vi "Playing with Resources.vi"() -> ()   [LabVIEW 2012]
uses:
  _ResManager_v86/ID_Resource info.ctl
  _ResManager_v86/IDCloneResMgr.lvlib
panel:
  out "Array":string[](array[string])
  in  "resource binary file":path=path "C:/Users/Francois/SkyDrive/_DESIM/Projets/UI Tools Addons/UI Tools Control Class/ctl_class/Templates/System vectoriel.ctl"
  out "resources":T1[](array[typedef]) {"type" format="%.0x"}
  out "file type":string
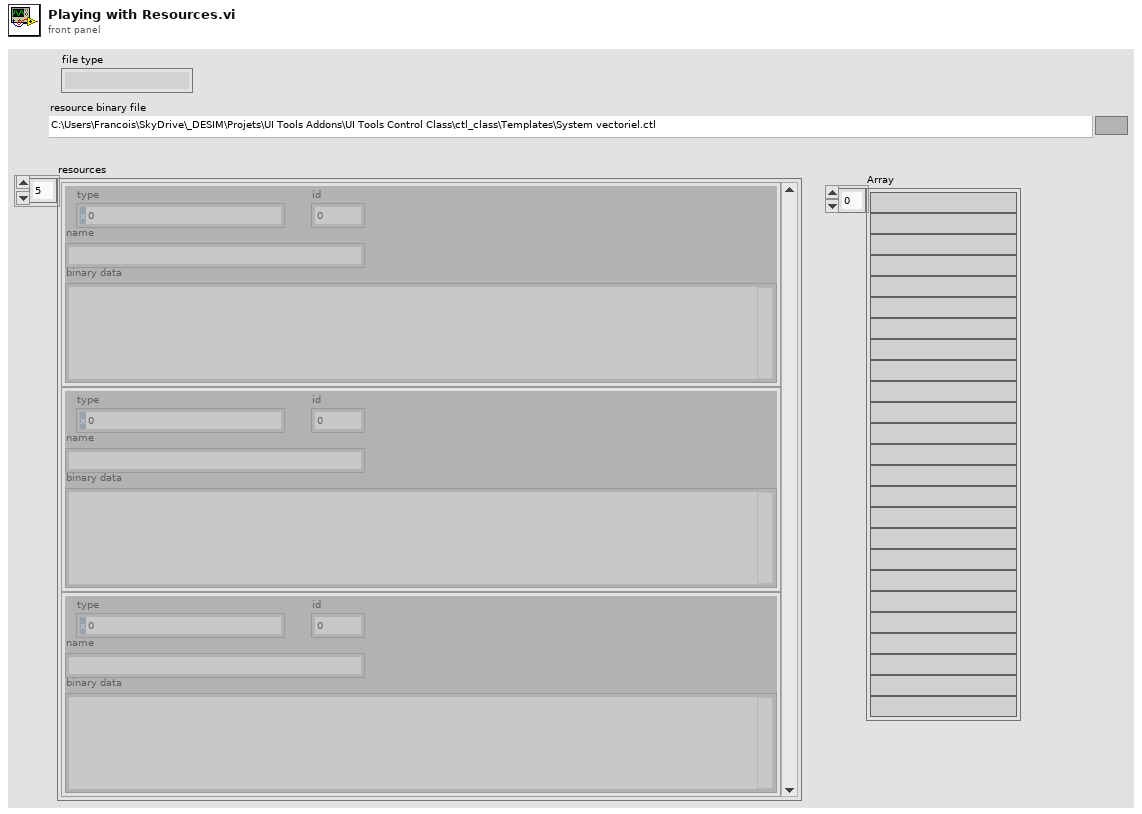
[diagram p1: front panel]
types:
  T1 = typedef "IDCloneResMgr.lvlib/ID_Resource info.ctl" = cluster{"type":u32, "id":i32, "name":string, "binary data":string}
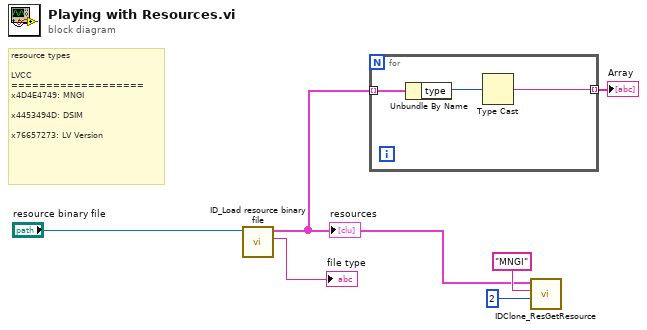
[diagram p0: block diagram]
diagram:
  # "resource types\n\nLVCC\n===================\nx4D4E4749: MNGI\n\nx4453494D: DSIM\n\nx76657273: LV Version"
  n1 = call "ID_Load resource binary file.vi"("resource binary file"="resource binary file") -> ("file type"=→"file type":string, "resources"=w2:T1[])  [unwired: 9 out]
  "resources" <- w2
  n2 = for {
    tunnel: w2 -> [w9] mode=indexing
    tunnel: [w7] -> w1 mode=indexing
    n3 = Unbundle By Name(w9) -> ("type"=w8:u32)
    n4 = Type Cast(x=w8) -> (*(type *) &x=w7:string)  [unwired: 1 in]
  }
  "Array" <- w1
  n5 = call "IDClone_ResGetResource.vi"("id"=2, "type"="MNGI" ("type string"), "resources"=w2) -> ()  [unwired: 1 in, 8 out]
